vi "Calc Velocity Setpoints.vi"(8 "v scale":dbl=1.0, 9 "Iterations":i32, 11 "Path stuff":T4 {"Limits"."Limits"."StoopidFast (fps)" min=0.0; "Limits"."Limits"."Jerk (fps^3)" min=0.0 step=1.0; "Limits"."Limits"."Accel (fps^2)" min=0.0; "Limits"."Limits"."Velocity (fps)" min=0.0}) -> (1 "tick count(ms)":u32, 2 "finished?":bool, 3 "setpoints":cluster{"left":dbl, "right":dbl})   [LabVIEW 2019]
uses:
  Support Code/Single Cmd Info.ctl
  <vilib>/picture/picture.llb/imagedata.ctl
  Support Code/types/Limits.ctl
  <vilib>/addons/control/pid/pid.llb/PID (DBL).vi
  <vilib>/addons/control/pid/NI_PID_pid.lvlib
panel:
  in  "i cant turn":dbl=1.0
  in  "ff":dbl=1.4
  in  "override":bool
  in  "Angle":dbl
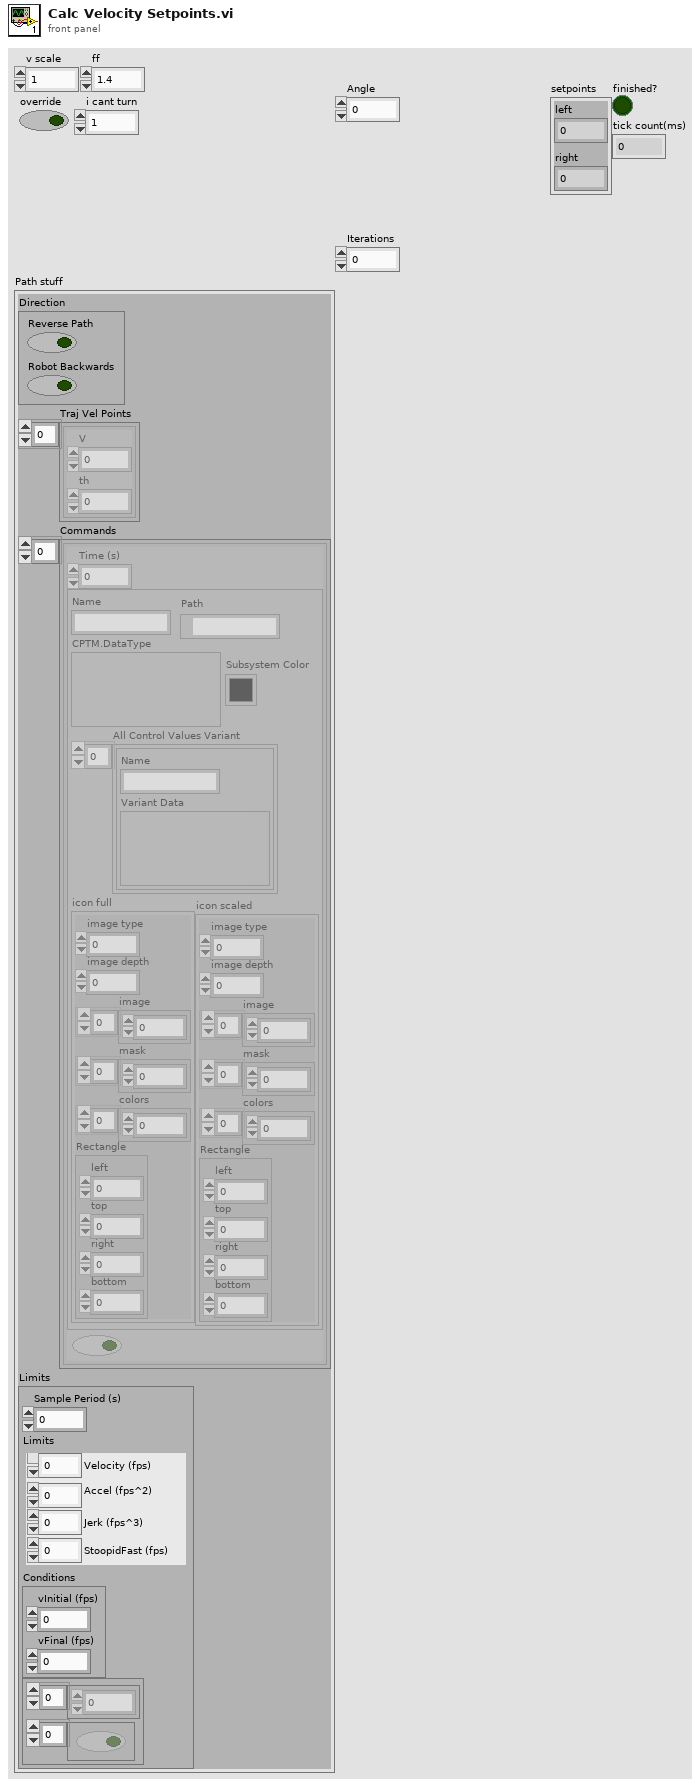
[diagram p1: front panel]
types:
  T1 = typedef "Single Cmd Info.ctl" = cluster{"Name":string, "CPTM.DataType":variant, "All Control Values Variant":cluster{"Name":string, "Variant Data":variant}[], "icon full":T2, "icon scaled":T2, "Path":path, "Subsystem Color":u32}
  T2 = typedef "imagedata.ctl" = cluster{"image type":i32, "image depth":i32, "image":u8[], "mask":u8[], "colors":u32[], "Rectangle":cluster{"left":i16, "top":i16, "right":i16, "bottom":i16}}
  T3 = typedef "Limits.ctl" = cluster{"Velocity (fps)":dbl, "Accel (fps^2)":dbl, "Jerk (fps^3)":dbl, "StoopidFast (fps)":dbl}
  T4 = cluster{"Direction":cluster{"Reverse Path":bool, "Robot Backwards":bool}, "Traj Vel Points":cluster{"V":dbl, "th":dbl}[], "Commands":cluster{"Time (s)":dbl, T1, bool}[], "Limits":cluster{"Sample Period (s)":dbl, "Limits":T3, "Conditions":cluster{"vInitial (fps)":dbl, "vFinal (fps)":dbl}, cluster{dbl[], bool[]}}}
  T5 = cluster{"Reverse Path":bool, "Robot Backwards":bool}
  T6 = cluster{"proportional gain (Kc)":dbl, "integral time (Ti, min)":dbl, "derivative time (Td, min)":dbl}
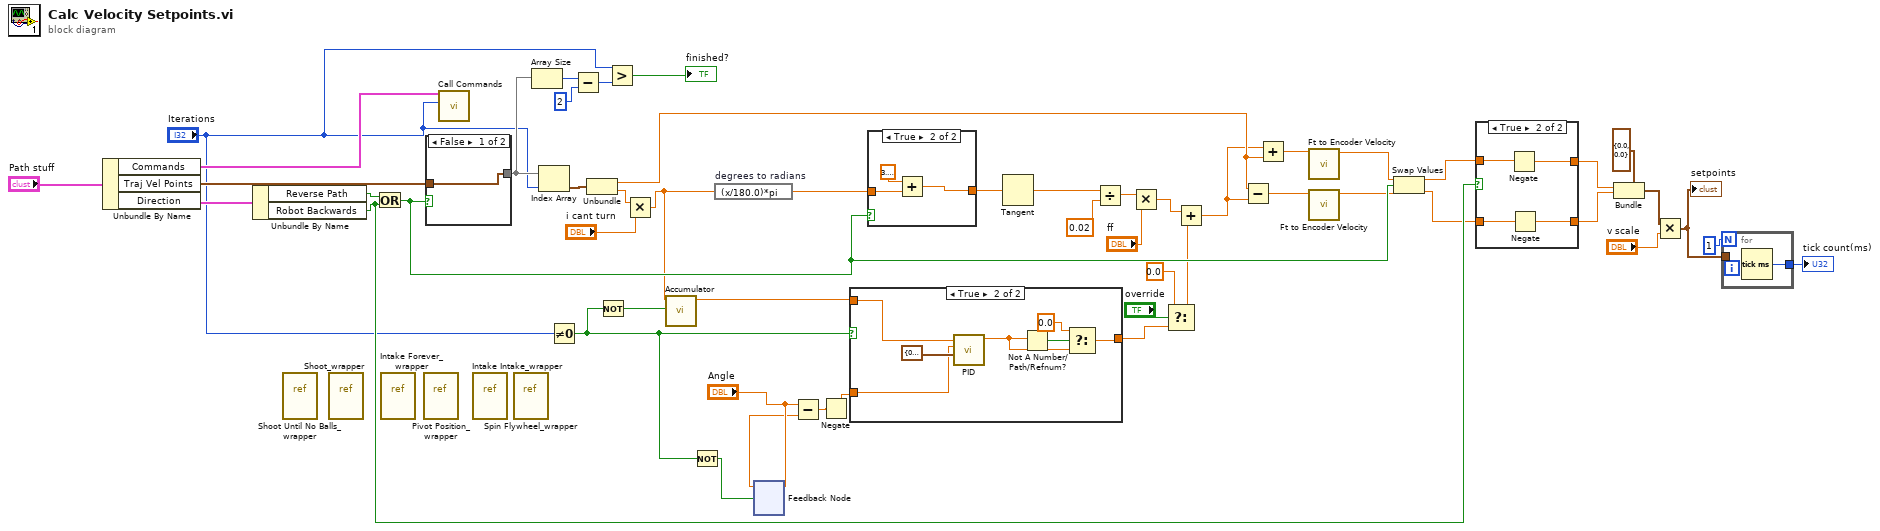
[diagram p0: block diagram]
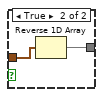
[diagram p4: hidden frame]
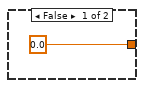
[diagram p5: hidden frame]
diagram:
  n1 = Unbundle By Name("Path stuff") -> ("Commands"=w52:cluster{"Time (s)":dbl, T1, bool}[], "Traj Vel Points"=w48:cluster{"V":dbl, "th":dbl}[], "Direction"=w50:T5)
  n2 = Unbundle By Name(w50) -> ("Reverse Path"=w49:bool, "Robot Backwards"=w35:bool)
  n3 = vi-ref "Shoot Until No Balls_wrapper.vi"() -> ()  [unwired: 1 out]
  n4 = vi-ref "Shoot_wrapper.vi"() -> ()  [unwired: 1 out]
  n5 = Or(x=w49, y=w35) -> (x .or. y?=w38:bool)
  n6 = vi-ref "Intake Forever_wrapper.vi"() -> ()  [unwired: 1 out]
  n7 = vi-ref "Pivot Position_wrapper.vi"() -> ()  [unwired: 1 out]
  n8 = case shown="False" w38 {
    tunnel: w48 -> [w53 w55]
    tunnel: [w53 w54] -> w29
    frame False {
    }
    frame True {
      n9 = Reverse 1D Array(array=w55) -> (reversed array=w54:cluster{"V":dbl, "th":dbl}[])
    }
  }
  n10 = call "Call Commands.vi"("Iterations"="Iterations", "Commands"=w52) -> ()  [unwired: 10 in]
  n11 = vi-ref "Intake Intake_wrapper.vi"() -> ()  [unwired: 1 out]
  n12 = vi-ref "Spin Flywheel_wrapper.vi"() -> ()  [unwired: 1 out]
  n13 = Array Size(array=w29) -> (size(s)=w28:i32)
  n14 = Index Array(array=w29, index="Iterations") -> (element=w47:cluster{"V":dbl, "th":dbl})
  n15 = Not Equal To 0?(x="Iterations") -> (x != 0?=w21:bool)
  n16 = Subtract(x=w28, y=2) -> (x-y=w26:i32)
  n17 = Unbundle(w47) -> ("V"=w41:dbl, "th"=w8:dbl)
  n18 = Not(x=w21) -> (.not. x?=w20:bool)
  n19 = Greater?(x="Iterations", y=w26) -> (0:→"finished?":bool)
  n20 = Multiply(x=w8, y="i cant turn") -> (x*y=w6:dbl)
  n21 = call "Accumulator.vi"("Reset?"=w20, "Value"=w6) -> ("Sum"=w19:dbl)  [unwired: 9 in]
  n22 = Not(x=w21) -> (.not. x?=w3:bool)
  n23 = expression code="(x/180.0)*pi" "degrees to radians"(w6) -> (w46:dbl)
  n24 = feedback-in #1("Angle", w3) -> ()
  n25 = feedback #1() -> (w1:dbl)  [unwired: 1 in]
  n26 = Subtract(x="Angle", y=w1) -> (x-y=w5:dbl)
  n27 = Negate(x=w5) -> (-x=w4:dbl)
  n28 = case shown="True" w21 {
    tunnel: w4 -> [_ w62]
    tunnel: w19 -> [_ w61]
    tunnel: [0.0 ("output") w57] -> w16
    frame False {
    }
    frame True {
      n29 = call-poly <vilib>:"PID.vi"("PID gains"=T6 {"proportional gain (Kc)"=0.08, "integral time (Ti, min)"=0.0, "derivative time (Td, min)"=0.001} ("PID gains L/S 2"), "process variable"=w62, "setpoint"=w61) -> ("output"=w59:dbl)  [unwired: 7 in, 1 out]
      n30 = Not A Number/Path/Refnum?(number/path/refnum=w59) -> (NaN/Path/Refnum?=w60:bool)
      n31 = Select(t=0.0, s=w60, f=w59) -> (s? t:f=w57:dbl)
    }
  }
  n32 = case shown="True" w38 {
    tunnel: w46 -> [w64 w67]
    tunnel: [w64 w65] -> w45
    frame False {
    }
    frame True {
      n33 = Add(x=3.141592653589793, y=w67) -> (x+y=w65:dbl)
    }
  }
  n34 = Tangent(1:w45) -> (0:w44:dbl)
  n35 = Divide(x=w44, y=0.02) -> (x/y=w42:dbl)
  n36 = Multiply(x=w42, y="ff") -> (x*y=w18:dbl)
  n37 = Select(t=0.0, s="override", f=w16) -> (s? t:f=w13:dbl)
  n38 = Add(x=w18, y=w13) -> (x+y=w17:dbl)
  n39 = Subtract(x=w41, y=w17) -> (x-y=w39:dbl)
  n40 = Add(x=w17, y=w41) -> (x+y=w40:dbl)
  n41 = call "Ft to Encoder Velocity.vi"("ft/s"=w40) -> ("v"=w37:dbl)  [unwired: 10 in]
  n42 = call "Ft to Encoder Velocity.vi"("ft/s"=w39) -> ("v"=w36:dbl)  [unwired: 10 in]
  n43 = Swap Values(12:w37, 13:w38, 14:w36) -> (1:w34:dbl, 3:w33:dbl)
  n44 = case shown="True" w35 {
    tunnel: w34 -> [w69 w73]
    tunnel: w33 -> [w68 w72]
    tunnel: [w69 w71] -> w31
    tunnel: [w68 w70] -> w30
    frame False {
    }
    frame True {
      n45 = Negate(x=w73) -> (-x=w71:dbl)
      n46 = Negate(x=w72) -> (-x=w70:dbl)
    }
  }
  n47 = Bundle(cluster=cluster{"left":dbl, "right":dbl} {"left"=0.0, "right"=0.0} ("setpoints"), "left"=w31, "right"=w30) -> (w23:cluster{"left":dbl, "right":dbl})
  n48 = Multiply(x=w23, y="v scale") -> (x*y=w11:cluster{"left":dbl, "right":dbl})
  "setpoints" <- w11
  n49 = for {
    N: 1 -> [_]
    tunnel: w11 -> [_]
    tunnel: [w74] -> w9
    n50 = Tick Count (ms)() -> (millisecond timer value=w74:u32)
  }
  "tick count(ms)" <- w9
